vi "拉氏变换.vi"() -> ()   [LabVIEW 2018]
uses:
  <vilib>/measure/NI_MABase.lvlib
  <vilib>/gmath/NI_Gmath.lvlib
panel:
  in  "停止":bool
  out "波形图 2":dbl[](graph)
  out "波形图":waveform(dbl)(graph)
  in  "频率":dbl(knob) scale=0.0..100.0
  in  "幅值":dbl(knob) scale=0.0..10.0
  in  "signal type":T1(ring) caption="信号类型"
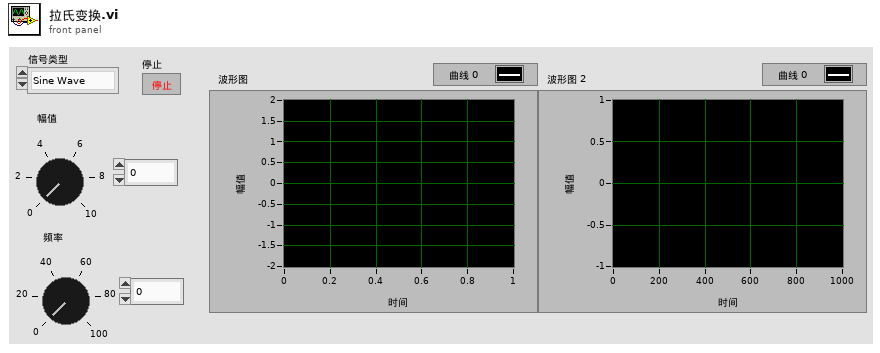
[diagram p1: front panel]
types:
  T1 = enum16{"Sine Wave", "Triangle Wave", "Square Wave", "Sawtooth Wave"}
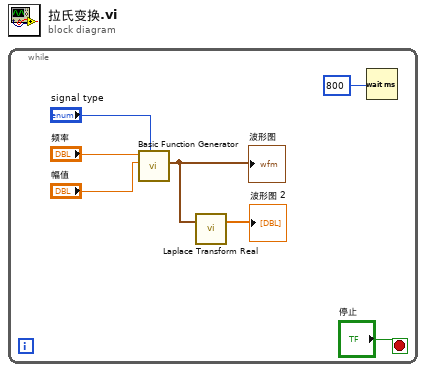
[diagram p0: block diagram]
diagram:
  n1 = while {
    stop <- "停止" stop-if-true
    n2 = call <vilib>:"Basic Function Generator.vi"("signal type"="signal type", "amplitude"="幅值", "frequency"="频率") -> ("signal out"=w4:waveform(dbl))  [unwired: 6 in, 2 out]
    "波形图" <- w4
    n3 = call <vilib>:"Laplace Transform Real.vi"("X"=w4) -> ("Laplace {X}"=→"波形图 2":dbl[])  [unwired: 1 in, 1 out]
    n4 = Wait (ms)(milliseconds to wait=u32 800 ("毫秒计时值")) -> ()  [unwired: 1 out]
  }
